vi "MM6.ReadXml.vi"(0 "i ref in":refnum<vi>, 1 "Data":string, 3 "timeout ms":i32=10000, 5 "error in (no error)":errorcluster) -> (14 "i ref out":refnum<vi>, 17 "timed out":bool, 19 "error out":errorcluster)   [LabVIEW 2014, in "MM6.lvlib"]
doc: "This method converts the raw XML string into \"ConfigData\" and writes this data to the attributes."
uses:
  MM6.lvlib
  LEBITDefs/LEBITDefs.ConfigData.ctl
  LEBITDefs/LEBITDefs.GenConfig.ctl
  LEBITDefs/LEBITDefs.Log.ctl
  LEBITDefs/LEBITDefs.OneConfig.ctl
  LEBITDefs/LEBITDefs.MCA.ctl
  LEBITDefs/LEBITDefs.Timing.ctl
  LEBITDefs/LEBITDefs.Timetable.ctl
  LEBITDefs/LEBITDefs.Memory.ctl
  LEBITDefs/LEBITDefs.ScanDev.ctl
  LEBITDefs/LEBITDefs.FreqDev.ctl
  LEBITDefs/LEBITDefs.CleanDev.ctl
  LEBITDefs/LEBITDefs.CleanDataType.ctl
  LEBITDefs/LEBITDefs.Special.ctl
  LEBITDefs/LEBITDefs.Delay.ctl
  LEBITDefs/LEBITDefs.DAC.ctl
  LEBITDefs/LEBITDefs.lvlib
panel:
  in  "Configs":T1[](array[typedef])=[{"MCA"={"Name"="SimMCS", "Address"="", "NrChannels"=1024, "Gate"=3, "NrPipse"=1}, "Timing"={"TimeTables"=[{"TimeTable"=[100.0, 200.0, 150.0]}], "Memories"=[{"Device"="SimTG", "ExtTrig"=FALSE, "TT2Use"=0, "PatternTable"=["aAa", "abC", "bBb", "cCc", "abC"]}], "ScanX"="", "ScanY"=""}, "Scans"=[{"Name"="SimAFG", "FctName"="SetFrequency", "Values"=[0.0, 1.0, 2.0, 3.0, 4.0], "NrScanVals"=5, "Special"=""}, {"Name"="*", "FctName"="*", "Values"=[1.0], "NrScanVals"=1, "Special"="*"}], "FreqDevs"=[{"Name"="SimAFG", "Amp"=1.0, "CenterFreq"=12345.0, "Time"=0.9}], "CleanDev"={"Name"="*Ooohhhh", "CleanData"=[{"Amp"=0.001, "Center"=5.0, "Plus"=1.0, "Minus"=1.0, "Time"=0.6}]}, "NrCycles"=17, "Specials"=[], "Delays"=[], "DAC"={"Name"="", "Step1"=0, "Step2"=0}}] {"CleanDev"."CleanData"."Time" format="%.3f"; "CleanDev"."CleanData"."Minus" format="%.2f"; "CleanDev"."CleanData"."Plus" format="%.2f"; "CleanDev"."CleanData"."Center" format="%.4f"; "CleanDev"."CleanData"."Amp" format="%.2f"; "Delays"."Delay" format="%.2f"; "Specials"."Data" format="%.2f"; "FreqDevs"."Time" format="%.3f"; "FreqDevs"."CenterFreq" format="%.4f"; "FreqDevs"."Amp" format="%.2f"; "Scans"."Values" format="%.2f"}
  in  "ConfigData":T13 {"Configs"."CleanDev"."CleanData"."Time" format="%.3f"; "Configs"."CleanDev"."CleanData"."Minus" format="%.2f"; "Configs"."CleanDev"."CleanData"."Plus" format="%.2f"; "Configs"."CleanDev"."CleanData"."Center" format="%.4f"; "Configs"."CleanDev"."CleanData"."Amp" format="%.2f"; "Configs"."Delays"."Delay" format="%.2f"; "Configs"."Specials"."Data" format="%.2f"; "Configs"."FreqDevs"."Time" format="%.3f"; "Configs"."FreqDevs"."CenterFreq" format="%.4f"; "Configs"."FreqDevs"."Amp" format="%.2f"; "Configs"."Scans"."Values" format="%.2f"}
  # "for testing purposes"
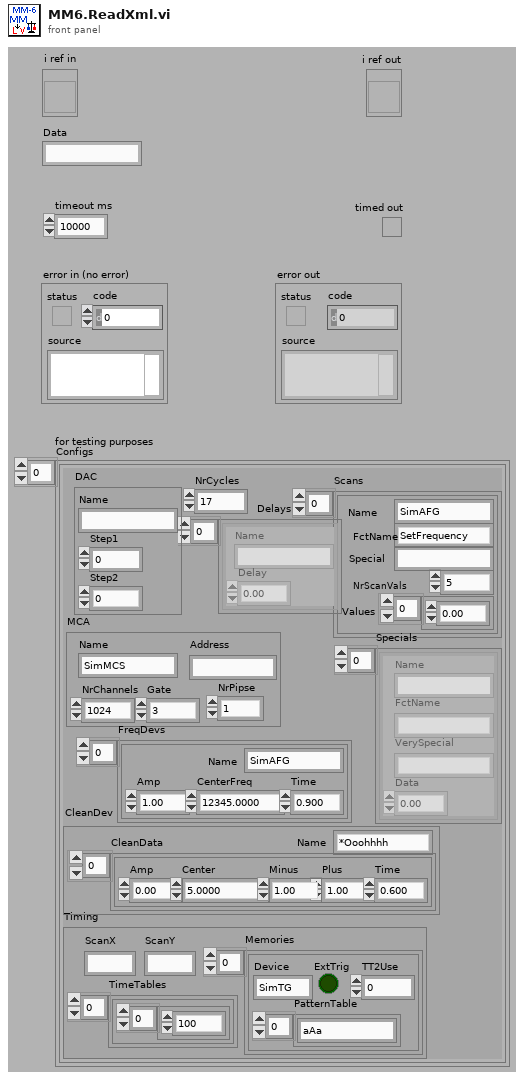
[diagram p1: front panel]
types:
  T1 = typedef "LEBITDefs.lvlib/LEBITDefs.OneConfig.ctl" = cluster{"MCA":T2, "Timing":T3, "Scans":T6[], "FreqDevs":T7[], "CleanDev":T8, "NrCycles":i32, "Specials":T10[], "Delays":T11[], "DAC":T12}
  T2 = typedef "LEBITDefs.lvlib/LEBITDefs.MCA.ctl" = cluster{"Name":string, "Address":string, "NrChannels":i32, "Gate":i32, "NrPipse":i32}
  T3 = typedef "LEBITDefs.lvlib/LEBITDefs.Timing.ctl" = cluster{"TimeTables":cluster{"TimeTable":T4}[], "Memories":T5[], "ScanX":string, "ScanY":string}
  T4 = typedef "LEBITDefs.lvlib/LEBITDefs.Timetable.ctl" = dbl[]
  T5 = typedef "LEBITDefs.lvlib/LEBITDefs.Memory.ctl" = cluster{"Device":string, "ExtTrig":bool, "TT2Use":i32, "PatternTable":string[]}
  T6 = typedef "LEBITDefs.lvlib/LEBITDefs.ScanDev.ctl" = cluster{"Name":string, "FctName":string, "Values":dbl[], "NrScanVals":i32, "Special":string}
  T7 = typedef "LEBITDefs.lvlib/LEBITDefs.FreqDev.ctl" = cluster{"Name":string, "Amp":dbl, "CenterFreq":dbl, "Time":dbl}
  T8 = typedef "LEBITDefs.lvlib/LEBITDefs.CleanDev.ctl" = cluster{"Name":string, "CleanData":T9[]}
  T9 = typedef "LEBITDefs.lvlib/LEBITDefs.CleanDataType.ctl" = cluster{"Amp":dbl, "Center":dbl, "Plus":dbl, "Minus":dbl, "Time":dbl}
  T10 = typedef "LEBITDefs.lvlib/LEBITDefs.Special.ctl" = cluster{"Name":string, "FctName":string, "VerySpecial":string, "Data":dbl}
  T11 = typedef "LEBITDefs.lvlib/LEBITDefs.Delay.ctl" = cluster{"Name":string, "Delay":dbl}
  T12 = typedef "LEBITDefs.lvlib/LEBITDefs.DAC.ctl" = cluster{"Name":string, "Step1":i32, "Step2":i32}
  T13 = typedef "LEBITDefs.lvlib/LEBITDefs.ConfigData.ctl" = cluster{"GenConfig":T14, "Configs":T1[]}
  T14 = typedef "LEBITDefs.lvlib/LEBITDefs.GenConfig.ctl" = cluster{"Mode":i32, "Logs":T15[]}
  T15 = typedef "LEBITDefs.lvlib/LEBITDefs.Log.ctl" = cluster{"Name":string, "FctName":string, "Special":string}
  T16 = typedef "MM6.lvlib/MM6.i attribute.ctl" = cluster{"ConfigData":T13, "UsedObjs":string[], "ActScanStep":i32[], "AbortRequest":bool, "StopRequest":bool, "# cycles":i32, "Connected":bool, "MMStatus":T17, "# data":i32, "DIMServices":cluster{"MM6StatusString":string, "MM6StatusID":i32, "discArchiver":string, "discArchiverID":i32, "eventBuilder":string, "eventBuilderID":i32, "GUIIDString":string, "GUIIDStringID":i32}, "dataFile":string, "ExtraDataSets":T18, "PGRunning":T19}
  T17 = typedef "MM6.lvlib/MM6.status.ctl" = enum16{"loaded", "load_error", "config", "config_error", "init", "init_error", "data_reset", "data_reset_error", "running", "start_error", "run_error", "abort_requested", "aborted", "stop_requested", "stopped", "stop_error", "Connected", "NOTConnected"}
  T18 = typedef "LEBITDefs.lvlib/LEBITDefs.ExtraData.ctl" = cluster{"Ions":cluster{"ExcitIonMass":string, "ExcitIonCharge":i32, "CleanIons":cluster{"CleanIonMass":string, "CleanIonCharge":i32}[]}, "TimingDescription":cluster{"TimeTableDescription":cluster{"Times":string[]}[], "PatternTableDescription":cluster{"Pattern":string[]}[]}, "ScanUnits":string[]}[]
  T19 = typedef "PPG_ABC.lvlib/PPG_ABC.PG_Running.ctl" = i32
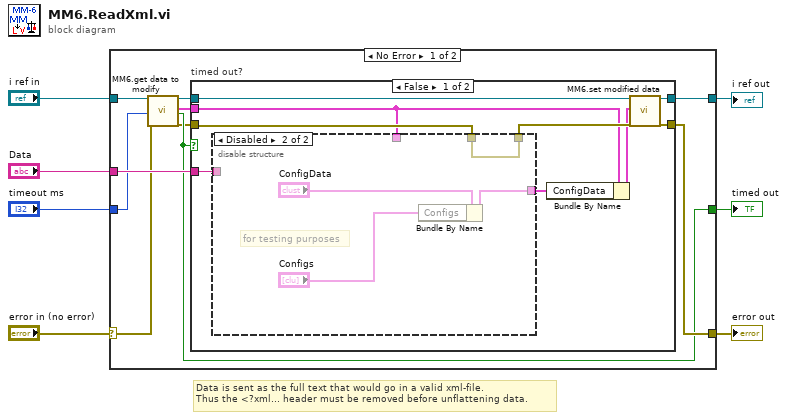
[diagram p0: block diagram]
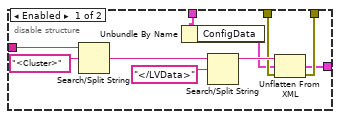
[diagram p2: hidden frame]
diagram:
  # "Data is sent as the full text that would go in a valid xml-file.\nThus the <?xml... header must be removed before unflattening data."
  n1 = case shown="No Error" "error in (no error)" {
    selector: "error in (no error)" -> [w13 w44]
    tunnel: [w17 w44] -> w7
    tunnel: "Data" -> [w16 _]
    tunnel: "i ref in" -> [w15 w43]
    tunnel: "timeout ms" -> [w14 _]
    tunnel: [w12 _] -> w2
    tunnel: [w9 w43] -> w1
    frame No Error {
      n2 = call "MM6.get data to modify.vi"("i ref in"=w15, "ms timeout (10000)"=w14, "error in (no error)"=w13) -> ("i ref out"=w10:refnum<vi>, "i attribute"=w8:T16, "timed out"=w12:bool, "error out"=w11:errorcluster)  [unwired: 13 in]
      n3 = case "timed out?" shown="False" w12 {
        tunnel: [w21 w42] -> w17
        tunnel: w16 -> [w26 _]
        tunnel: w11 -> [w25 w42]
        tunnel: w10 -> [w24 w41]
        tunnel: [w22 w41] -> w9
        tunnel: w8 -> [w18 _]
        frame False {
          n4 = disable-structure shown="Disabled" {
            disable-tunnel: w26 -> [w32 _]
            disable-tunnel: w25 -> [w31 w40]
            disable-tunnel: [w30 w40] -> w23
            disable-tunnel: [w29 w38] -> w19
            disable-tunnel: w18 -> [w28 _]
            frame Enabled {
              n5 = Search/Split String(string=w32, search string/char (-)="<Cluster>") -> (match + rest of string=w35:string)  [unwired: 1 in, 2 out]
              n6 = Unbundle By Name(w28) -> ("ConfigData"=w27:T13)
              n7 = Search/Split String(string=w35, search string/char (-)="</LVData>") -> (substring before match=w33:string)  [unwired: 1 in, 2 out]
              n8 = Unflatten From XML(xml string=w33, type=w27, error in (no error)=w31) -> (value=w29:T13, error out=w30:errorcluster)
            }
            frame Disabled {
              # "for testing purposes"
              n9 = Bundle By Name(cluster="ConfigData", "Configs"="Configs") -> (w38:T13)
            }
          }
          n10 = Bundle By Name(cluster=w18, "ConfigData"=w19) -> (w20:T16)
          n11 = call "MM6.set modified data.vi"("i ref in"=w24, "i attribute"=w20, "error in (no error)"=w23) -> ("i ref out"=w22:refnum<vi>, "error out"=w21:errorcluster)  [unwired: 15 in]
        }
        frame True {
        }
      }
    }
    frame Error {
    }
  }
  "error out" <- w7
  "i ref out" <- w1
  "timed out" <- w2
